vi "Guys version.vi"() -> ()   [LabVIEW 2014]
uses:
  <vilib>/Platform/TimedLoop/XDataNode/XDataNode.xnode
  <vilib>/Platform/TimedLoop/XDataNode/nitl_modes.ctl
  <vilib>/Platform/TimedLoop/XDataNode/XDNodeRunTimeDep.lvlib
  <vilib>/Platform/TimedLoop/XDataNode/wakeup.ctl
  <vilib>/Platform/TimedLoop/XDataNode/timing_clust.ctl
  <instrlib>/_niInstr/Streaming/v1/FPGA/niInstr Streaming v1 FPGA.lvlib
  DRAM FIFO/K7 DRAM FIFO.lvclass
  <vilib>/rvi/DataTransferAndStorage/Container/XNode/niFpgaContainer.xnode
  <vilib>/rvi/FIFO/Fifo_Resource/niFpgaFifoEmulationRefIn.vi
  <instrlib>/_niInstr/Basic Elements/v1/FPGA/niInstr Basic Elements v1 FPGA.lvlib
  <instrlib>/_niInstr/Memory/v1/FPGA/DRAM/Public/Timeslot Arbiter Configuration.ctl
  <instrlib>/_niInstr/Memory/v1/FPGA/DRAM/niInstr Memory DRAM v1 FPGA.lvclass
  FPGA_Controls/Acquisition FIFOs Cluster.ctl
  <vilib>/rvi/FIFO/Fifo_Resource/nirvififoEmulationWrite.vi
  <vilib>/rvi/interface/RandomDataEmulation/nirviRandomDataFpgaReadWriteTemplate.vi
  <instrlib>/_niInstr/Streaming/v1/Common/Stream State.ctl
  <instrlib>/_niInstr/Streaming/v1/Common/niInstr Streaming v1 Common.lvlib
panel:
  in  "stream.num samples 1":u64
  out "stream.state 1":T1
  out "stream.samples transferred 1":u64
  in  "stream.request state 1":T1
  out "stream.metadata 1":u64
  out "stream.metadata 0":u64
  in  "stream.request state 0":T1
  out "stream.samples transferred 0":u64
  out "stream.state 0":T1
  in  "stream.num samples 0":u64
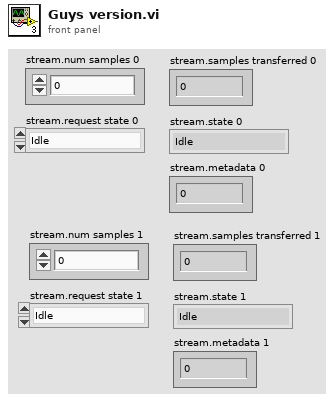
[diagram p1: front panel]
types:
  T1 = typedef "niInstr Streaming v1 Common.lvlib/Stream State.ctl" = enum8{"Idle", "Finite Transfer", "Continuous", "Done", "Error", "Not Ready", "Cancel"}
  T2 = typedef "Acquisition FIFOs Cluster.ctl" = cluster{"FIFO 0":refnum<k21>, "FIFO 1":refnum<k21>, "FIFO 2":refnum<k21>, "FIFO 3":refnum<k21>, "FIFO 4":refnum<k21>, "FIFO 5":refnum<k21>, "FIFO 6":refnum<k21>, "FIFO 7":refnum<k21>}
  T3 = typedef "XDNodeRunTimeDep.lvlib/timing_clust.ctl" = cluster{"Expected End [f-1]":u64, "Actual End [f-1]":u64, "Finished Late? [f-1]":bool, "Expected End [i-1]":u64, "Actual End [i-1]":u64, "Finished Late? [i-1]":bool, "Expected Start [i]":u64, "Actual Start [i]":u64, "Expected Start [f]":u64, "Actual Start [f]":u64, "Source Name":string, "Structure Name":string, "Period":i64, "Deadline":i64, "Offset":i64, "Start":i64, "Priority":i32, "Timeout":i32, "Mode":T4, "Wakeup Reason":T5, "Error":errorcluster, "Source Type":string, "Secondary Source Type":string, "Global End Time":u64, "Global Start Time":u64, "Frame Duration":u64, "Iteration Duration":u64, "Assigned CPU":i32, "I/O Scan Engine Mode":u32}
  T4 = typedef "XDNodeRunTimeDep.lvlib/nitl_modes.ctl" = enum32{"No Change", "Process missed periods, maintain original phase", "Discard missed periods, maintain original phase", "Process missed periods, ignore original phase", "Discard missed periods, ignore original phase"}
  T5 = typedef "XDNodeRunTimeDep.lvlib/wakeup.ctl" = enum32{"Normal", "Aborted", "Asynchronous wakeup", "Timing source error", "Timed loop error", "Timeout"}
  T6 = typedef "niInstr Memory DRAM v1 FPGA.lvclass/Timeslot Arbiter Configuration.ctl" = cluster{"write grant time (clocks)":u16, "read grant time (clocks)":u16}
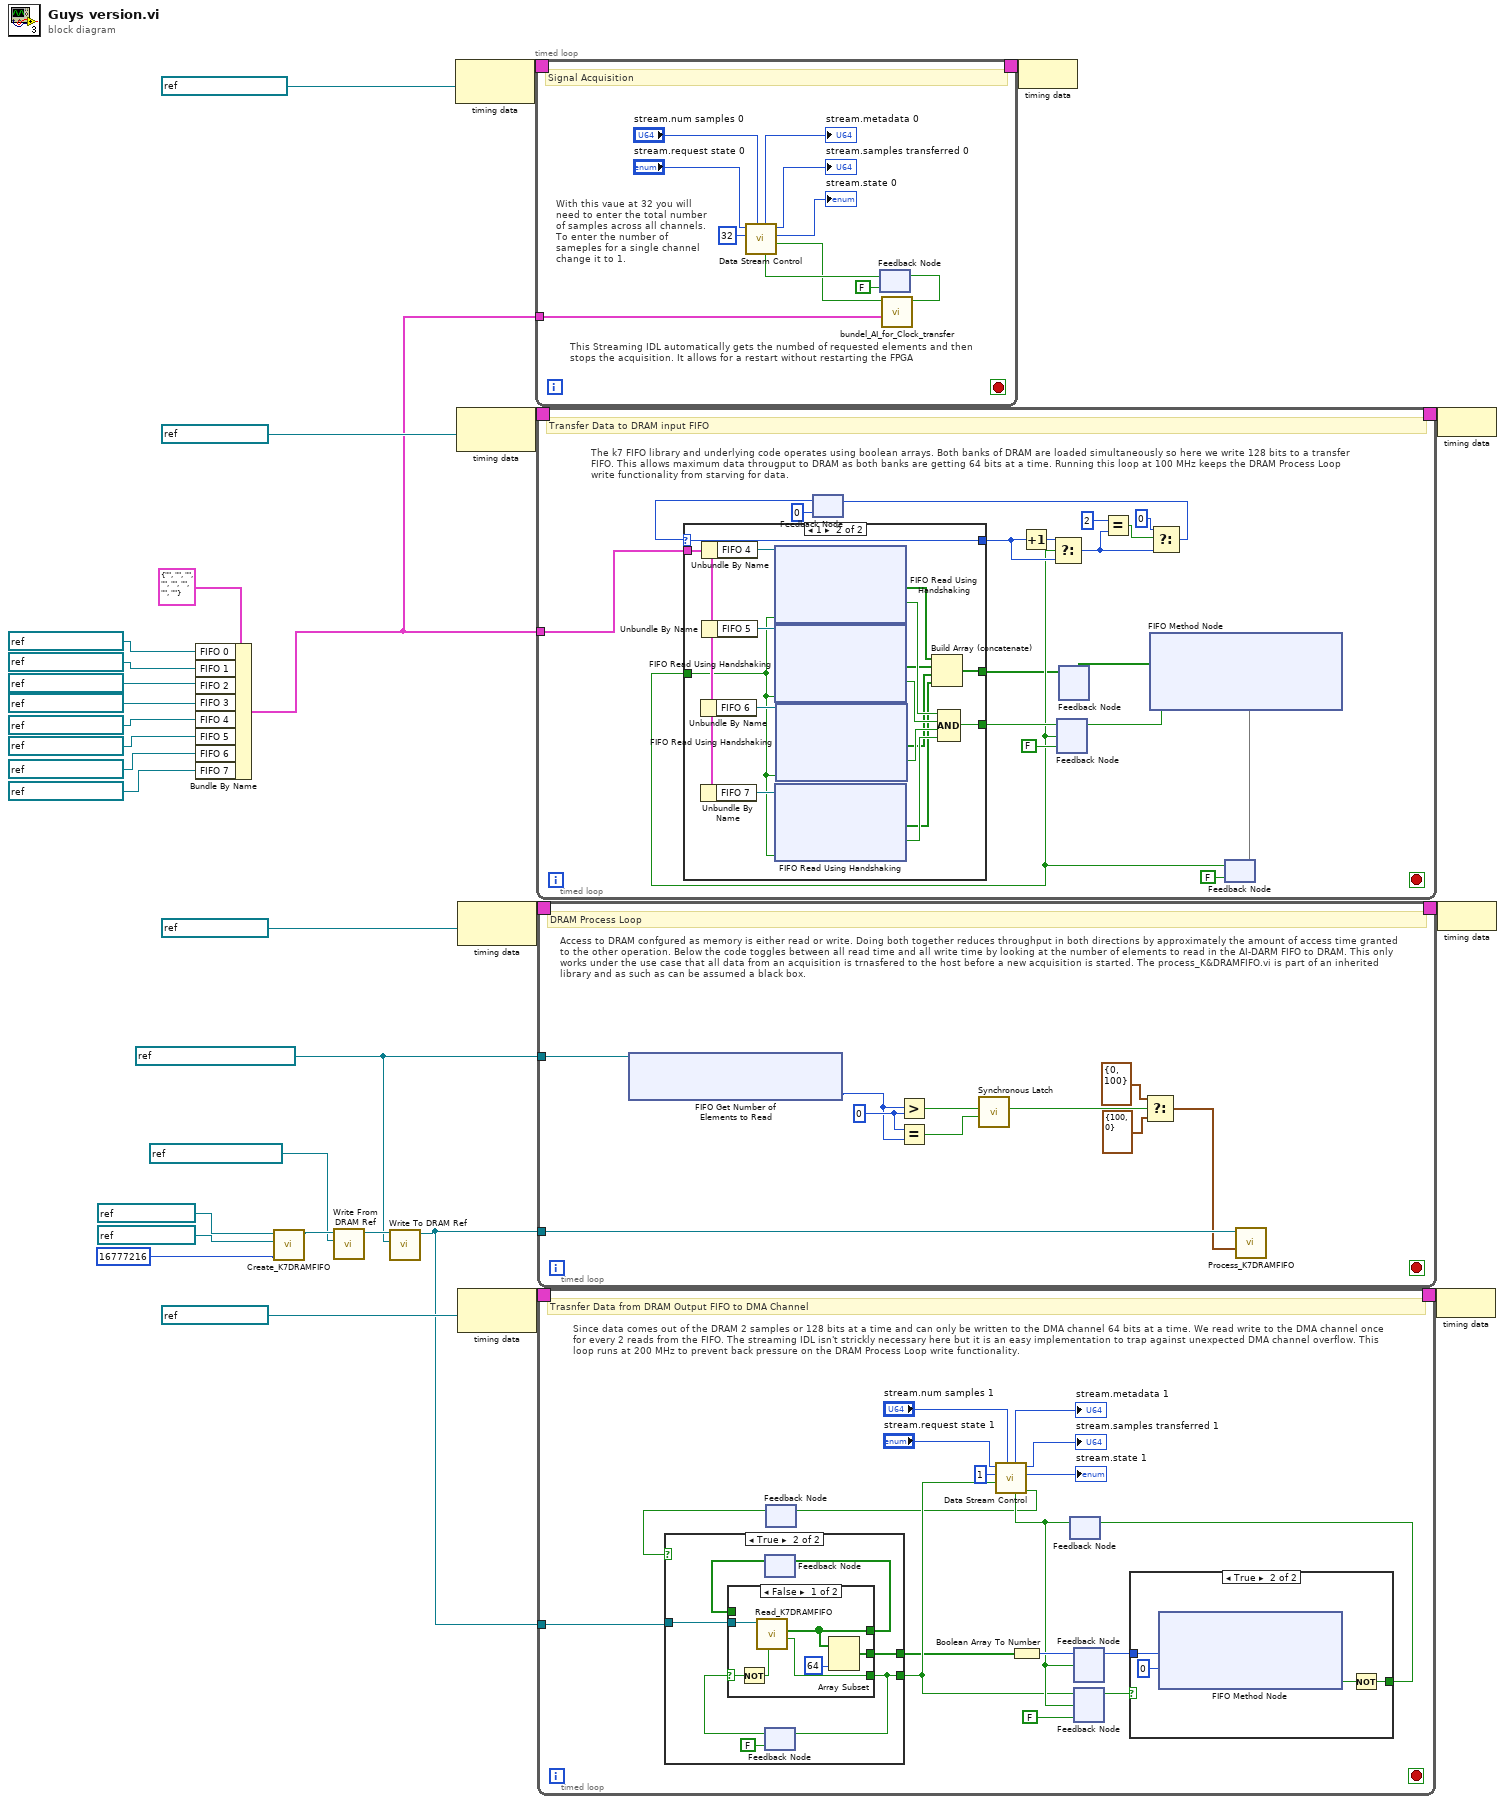
[diagram p0: block diagram]
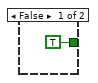
[diagram p2: hidden frame]
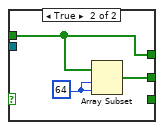
[diagram p4: hidden frame]
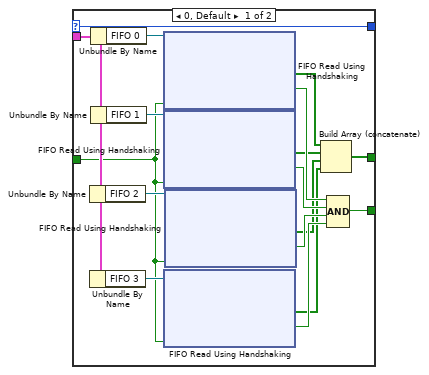
[diagram p5: hidden frame]
diagram:
  w2 = refnum<k21> "Bundeling to DRAM FIFO" ("FIFO In")
  n1 = Bundle By Name(cluster=T2 {"FIFO 0"="", "FIFO 1"="", "FIFO 2"="", "FIFO 3"="", "FIFO 4"="", "FIFO 5"="", "FIFO 6"="", "FIFO 7"=""} ("FIFO Refs"), "FIFO 0"=refnum<k21> "AI Bundel FIFO 0" ("FIFO In"), "FIFO 1"=refnum<k21> "AI Bundel FIFO 1" ("FIFO In"), "FIFO 2"=refnum<k21> "AI Bundel FIFO 2" ("FIFO In"), "FIFO 3"=refnum<k21> "AI Bundel FIFO 3" ("FIFO In"), "FIFO 4"=refnum<k21> "AI Bundel FIFO 4" ("FIFO In"), "FIFO 5"=refnum<k21> "AI Bundel FIFO 5" ("FIFO In"), "FIFO 6"=refnum<k21> "AI Bundel FIFO 6" ("FIFO In"), "FIFO 7"=refnum<k21> "AI Bundel FIFO 7" ("FIFO In")) -> (w18:T2)
  n2 = call "Create_K7DRAMFIFO.vi"("Requested # of Elements"=u32 16777216, "DRAM Bank 2 Ref"=refnum<k21> "DRAM FIFO 2" ("Memory In"), "DRAM Bank 1 Ref"=refnum<k21> "DRAM FIFO 1" ("Memory In")) -> ("DRAM FIFO Ref Out"=w14:refnum<class "K7 DRAM FIFO.lvclass">)  [unwired: 8 in]
  n3 = call "Write From DRAM Ref.vi"("From DRAM"=refnum<k21> "DRAM to DMA", "K7 DRAM FIFO in"=w14) -> ("K7 DRAM FIFO out"=w17:refnum<class "K7 DRAM FIFO.lvclass">)  [unwired: 9 in]
  n4 = call "Write To DRAM Ref.vi"("To DRAM"=w2, "K7 DRAM FIFO in"=w17) -> ("K7 DRAM FIFO out"=w16:refnum<class "K7 DRAM FIFO.lvclass">)  [unwired: 9 in]
  n5 = node-c288(refnum<k21> "IO Module Clock 0" ("Source Name")) -> (w30:T3)
  n6 = node-c288(refnum<k21> "100 MHz Clock" ("Source Name")) -> (w27:T3)
  n7 = node-c288(refnum<k21> "100 MHz Clock" ("Source Name")) -> (w24:T3)
  n8 = node-c288(refnum<k21> "200 MHz Clock" ("Source Name")) -> (w21:T3)
  n9 = timed-loop {
    timing: w30 -> [_]
    timing-out: [_] -> w29
    tunnel: w18 -> [w31]
    stop <- _ stop-if-true
    # "With this vaue at 32 you will need to enter the total number of samples across all channels. To enter the number of sameples for a single channel change it to 1."
    # "This Streaming IDL automatically gets the numbed of requested elements and then stops the acquisition. It allows for a restart without restarting the FPGA"
    # "Signal Acquisition"
    n10 = feedback #1(FALSE ("Ready for Input")) -> (w33:bool)
    n11 = call <instrlib>:"Data Stream Control.vi"("ready for input?"=w33, "stream.num samples 0"="stream.num samples 0", "element count"=u16 32, "stream.request state 0"="stream.request state 0") -> ("send data"=w32:bool, "stream.state 0"=→"stream.state 0":T1, "stream.samples transferred 0"=→"stream.samples transferred 0":u64, "stream.metadata 0"=→"stream.metadata 0":u64)  [unwired: 3 in, 1 out]
    n12 = call "bundel_AI_for_Clock_transfer.vi"("FIFO Refs"=w31, "Input Valid"=w32) -> ("Ready for Input"=w41:bool)  [unwired: 9 in]
    n13 = feedback-in #1(w41) -> ()
  }
  n14 = timed-loop {
    timing: w27 -> [_]
    timing-out: [_] -> w26
    tunnel: w18 -> [w61]
    stop <- _ stop-if-true
    # "The k7 FIFO library and underlying code operates using boolean arrays. Both banks of DRAM are loaded simultaneously so here we write 128 bits to a transfer FIFO. This allows maximum data througput to DRAM as both banks are getting 64 bits at a time. Running this loop at 100 MHz keeps the DRAM Process Loop write functionality from starving for data."
    # "Transfer Data to DRAM input FIFO"
    n15 = feedback #2(i16 0 ("t")) -> (w60:i16)
    n16 = feedback #3(FALSE ("Output Valid")) -> (w46:bool)
    n17 = feedback #4() -> (w44:bool[])  [unwired: 1 in]
    n18 = xnode ("FIFO Method Node")("Element"=w44, "Input Valid"=w46) -> ("Ready for Input"=w45)  [unwired: 1 in, 1 out]
    n19 = feedback-in #5(w45) -> ()
    n20 = feedback #5(FALSE ("Ready for Input")) -> (w54:bool)
    n21 = case shown="1" w60 {
      selector: w60 -> [w77 w94]
      tunnel: w61 -> [w63 w80]
      tunnel: [w75 w92] -> w47
      tunnel: [w68 w85] -> w59
      tunnel: [w77 w94] -> w55
      tunnel: w54 -> [w62 w79]
      frame 0, Default {
        n22 = Unbundle By Name(w63) -> ("FIFO 2"=w74:refnum<k21>)
        n23 = Unbundle By Name(w63) -> ("FIFO 3"=w73:refnum<k21>)
        n24 = Unbundle By Name(w63) -> ("FIFO 0"=w78:refnum<k21>)
        n25 = Unbundle By Name(w63) -> ("FIFO 1"=w76:refnum<k21>)
        n26 = xnode ("FIFO Read Using Handshaking")("Ready for Output"=w62, "FIFO In"=w78) -> ("Element"=w67:bool[], "Output Valid"=w72:bool)  [unwired: 1 out]
        n27 = xnode ("FIFO Read Using Handshaking")("Ready for Output"=w62, "FIFO In"=w76) -> ("Element"=w66:bool[], "Output Valid"=w71:bool)  [unwired: 1 out]
        n28 = xnode ("FIFO Read Using Handshaking")("Ready for Output"=w62, "FIFO In"=w73) -> ("Element"=w64:bool[], "Output Valid"=w69:bool)  [unwired: 1 out]
        n29 = xnode ("FIFO Read Using Handshaking")("Ready for Output"=w62, "FIFO In"=w74) -> ("Element"=w65:bool[], "Output Valid"=w70:bool)  [unwired: 1 out]
        n30 = Build Array (concatenate)(w67, w66, w65, w64) -> (w75:bool[])
        n31 = Compound Arithmetic op=AND(w72, w71, w70, w69) -> (w68:bool)
      }
      frame 1 {
        n32 = Unbundle By Name(w80) -> ("FIFO 6"=w91:refnum<k21>)
        n33 = Unbundle By Name(w80) -> ("FIFO 7"=w90:refnum<k21>)
        n34 = Unbundle By Name(w80) -> ("FIFO 4"=w95:refnum<k21>)
        n35 = Unbundle By Name(w80) -> ("FIFO 5"=w93:refnum<k21>)
        n36 = xnode ("FIFO Read Using Handshaking")("Ready for Output"=w79, "FIFO In"=w95) -> ("Element"=w84:bool[], "Output Valid"=w89:bool)  [unwired: 1 out]
        n37 = xnode ("FIFO Read Using Handshaking")("Ready for Output"=w79, "FIFO In"=w93) -> ("Element"=w83:bool[], "Output Valid"=w88:bool)  [unwired: 1 out]
        n38 = xnode ("FIFO Read Using Handshaking")("Ready for Output"=w79, "FIFO In"=w90) -> ("Element"=w81:bool[], "Output Valid"=w86:bool)  [unwired: 1 out]
        n39 = xnode ("FIFO Read Using Handshaking")("Ready for Output"=w79, "FIFO In"=w91) -> ("Element"=w82:bool[], "Output Valid"=w87:bool)  [unwired: 1 out]
        n40 = Build Array (concatenate)(w84, w83, w82, w81) -> (w92:bool[])
        n41 = Compound Arithmetic op=AND(w89, w88, w87, w86) -> (w85:bool)
      }
    }
    n42 = Increment(x=w55) -> (x+1=w56:i16)
    n43 = Select(t=w56, s=w54, f=w55) -> (s? t:f=w52:i16)
    n44 = feedback-in #3(w59, w54) -> ()
    n45 = feedback-in #4(w47) -> ()  [unwired: 1 in]
    n46 = Equal?(x=i16 2, y=w52) -> (x = y?=w51:bool)
    n47 = Select(t=i16 0, s=w51, f=w52) -> (s? t:f=w50:i16)
    n48 = feedback-in #2(w50) -> ()
  }
  n49 = timed-loop {
    timing: w24 -> [_]
    timing-out: [_] -> w23
    tunnel: w16 -> [w107]
    tunnel: w2 -> [w99]
    stop <- _ stop-if-true
    w103 = u32 0 ("x")
    # "Access to DRAM confgured as memory is either read or write. Doing both together reduces throughput in both directions by approximately the amount of access time granted to the other operation. Below the code toggles between all read time and all write time by looking at the number of elements to read in the AI-DARM FIFO to DRAM. This only works under the use case that all data from an acquisition is trnasfered to the host before a new acquisition is started. The process_K&DRAMFIFO.vi is part of an inherited library and as such as can be assumed a black box."
    # "DRAM Process Loop"
    n50 = xnode ("FIFO Get Number of Elements to Read")("FIFO In"=w99) -> ("Number of Elements to Read"=w98:u32)  [unwired: 1 out]
    n51 = Greater?(x=w98, y=w103) -> (0:w104:bool)
    n52 = Equal?(x=w103, y=w98) -> (x = y?=w102:bool)
    n53 = call <instrlib>:"Synchronous Latch.vi"("clear"=w102, "set"=w104) -> ("out"=w101:bool)  [unwired: 9 in]
    n54 = Select(t=T6 {"write grant time (clocks)"=0, "read grant time (clocks)"=100} ("arbiter configuration"), s=w101, f=T6 {"write grant time (clocks)"=100, "read grant time (clocks)"=0} ("arbiter configuration")) -> (s? t:f=w100:T6)
    n55 = call "Process_K7DRAMFIFO.vi"("arbiter configuration"=w100, "DRAM FIFO Ref In"=w107) -> ()  [unwired: 10 in]
  }
  n56 = timed-loop {
    timing: w21 -> [_]
    timing-out: [_] -> w20
    tunnel: w16 -> [w126]
    stop <- _ stop-if-true
    # "Since data comes out of the DRAM 2 samples or 128 bits at a time and can only be written to the DMA channel 64 bits at a time. We read write to the DMA channel once for every 2 reads from the FIFO. The streaming IDL isn't strickly necessary here but it is an easy implementation to trap against unexpected DMA channel overflow. This loop runs at 200 MHz to prevent back pressure on the DRAM Process Loop write functionality."
    # "Trasnfer Data from DRAM Output FIFO to DMA Channel"
    n57 = feedback #6() -> (w113:bool)  [unwired: 1 in]
    n58 = case shown="True" w113 {
      tunnel: w126 -> [_ w138]
      tunnel: [_ w136] -> w115
      tunnel: [_ w132] -> w112
      frame False {
      }
      frame True {
        n59 = feedback #7() -> (w137:bool[])  [unwired: 1 in]
        n60 = feedback #8(FALSE ("Output Valid")) -> (w135:bool)
        n61 = case shown="False" w135 {
          selector: w135 -> [w140 _]
          tunnel: w138 -> [w145 _]
          tunnel: [w143 w146] -> w133
          tunnel: w137 -> [_ w146]
          tunnel: [w144 _] -> w136
          tunnel: [w141 w148] -> w132
          frame False {
            n62 = Not(x=w140) -> (.not. x?=w139:bool)
            n63 = call "Read_K7DRAMFIFO.vi"("Ready for Output"=w139, "DRAM FIFO Ref In"=w145) -> ("Output Valid"=w144:bool, "Element"=w143:bool[])  [unwired: 7 in, 1 out]
            n64 = Array Subset(array=w143, length=64) -> (w141:bool[])  [unwired: 1 in]
          }
          frame True {
            w147 = 64 ("length")
            n65 = Array Subset(array=w146, index=w147, length=w147) -> (w148:bool[])
          }
        }
        n66 = feedback-in #7(w133) -> ()
        n67 = feedback-in #8(w136) -> ()
      }
    }
    n68 = Boolean Array To Number(Boolean array=w112) -> (number=w125:u64)
    n69 = feedback #9() -> (w116:bool)  [unwired: 1 in]
    n70 = call <instrlib>:"Data Stream Control.vi"("ready for input?"=w116, "stream.num samples 0"="stream.num samples 1", "data valid"=w115, "element count"=u16 1, "stream.request state 0"="stream.request state 1") -> ("request data"=w114:bool, "stream.state 0"=→"stream.state 1":T1, "stream.samples transferred 0"=→"stream.samples transferred 1":u64, "stream.metadata 0"=→"stream.metadata 1":u64)  [unwired: 2 in, 1 out]
    n71 = feedback-in #6(w114) -> ()
    n72 = feedback-in #10(w125, w116) -> ()
    n73 = feedback #10() -> (w124:u64)  [unwired: 1 in]
    n74 = feedback #11(FALSE ("Output Valid")) -> (w110:bool)
    n75 = feedback-in #11(w115, w116) -> ()
    n76 = case shown="True" w110 {
      tunnel: w124 -> [_ w131]
      tunnel: [TRUE w129] -> w111
      frame False {
      }
      frame True {
        n77 = xnode ("FIFO Method Node")("Element"=w131, "Timeout"=0) -> ("Timed Out?"=w130:bool)  [unwired: 1 in, 1 out]
        n78 = Not(x=w130) -> (.not. x?=w129:bool)
      }
    }
    n79 = feedback-in #9(w111) -> ()
  }
  n80 = node-c288(w29) -> ()
  n81 = node-c288(w20) -> ()
  n82 = node-c288(w26) -> ()
  n83 = node-c288(w23) -> ()
